vi "lua_monitor.vi"(11 "Lua for LabVIEW.lvlib:Lua.lvclass":refnum<data-value>) -> ()   [LabVIEW 2020, in "Lua for LabVIEW.lvlib" / "Lua.lvclass"]
uses:
  Lua.lvclass
  Lua.lvclass/Lua.ctl
  lib/lua.dll/lua.dll.lvlib
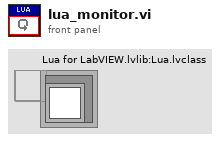
[diagram p1: front panel]
types:
  T1 = typedef "Lua for LabVIEW.lvlib/Lua.lvclass/lua_monitor_event.ctl" = enum16{"<null>", "terminate"}
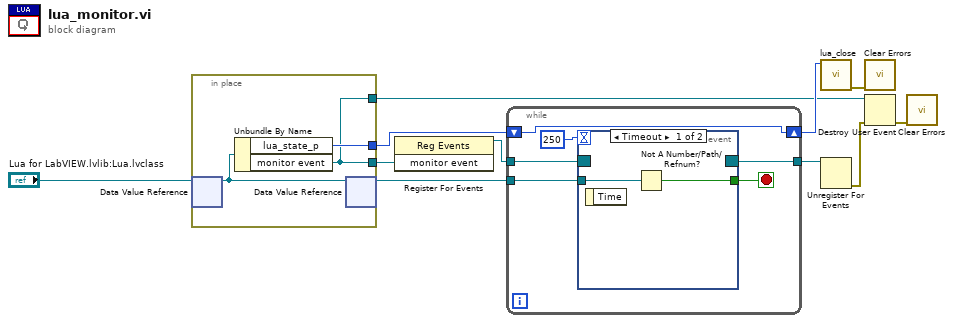
[diagram p0: block diagram]
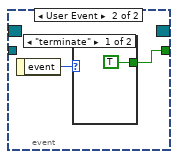
[diagram p2: hidden frame]
diagram:
  n1 = in-place {
    in-place-border: [w13] -> w8
    in-place-border: [w12] -> w2
    in-place-border: [w12] -> w7
    n2 = in-place-dvr #1("Lua for LabVIEW.lvlib:Lua.lvclass") -> (w14:refnum<class "Lua.lvclass">)  [unwired: 1 out]
    n3 = Unbundle By Name(w14) -> ("lua_state_p"=w13:u64, "monitor event"=w12:refnum<user-event>)
    n4 = in-place-dvr #1(w14) -> (w10:refnum<data-value>)  [unwired: 1 out]
  }
  n5 = register-events(w7) -> (reference out=w9:refnum<event-registration>)  [unwired: 2 in, 1 out]
  n6 = while {
    tunnel: w10 -> [w18]
    tunnel: w9 -> [w20]
    shift-right: [w16] -> w6
    shift-left: w8 -> [w16]
    tunnel: [w15] -> w4
    stop <- w17 stop-if-true
    n7 = event shown="[0] Timeout" {
      selector: w20 -> [_ _]
      dyn-events: [_ _] -> w15
      timeout: 250 -> [_ _]
      tunnel: w18 -> [w22 _]
      tunnel: [w21 w23] -> w17
      event Timeout {
        n8 = event-data() -> ()  [unwired: 1 in, 1 out]
        n9 = Not A Number/Path/Refnum?(number/path/refnum=w22) -> (NaN/Path/Refnum?=w21:bool)
      }
      event User Event {
        n10 = event-data() -> ("event"=w24:T1)  [unwired: 1 in]
        n11 = case shown="\"terminate\"" w24 {
          tunnel: [TRUE _] -> w23
          frame "terminate" {
          }
          frame Default {
          }
        }
      }
    }
  }
  n12 = call "lua_close.vi"("lua_state_p"=w6) -> ("error out"=w5:errorcluster)  [unwired: 10 in]
  n13 = Unregister For Events(event registration refnum=w4) -> (error out=w3:errorcluster)  [unwired: 1 in]
  n14 = call <vilib>:"Clear Errors.vi"("error in (no error)"=w5) -> ()  [unwired: 5 in, 2 out]
  n15 = Destroy User Event(user event=w2, error in=w3) -> (error out=w1:errorcluster)
  n16 = call <vilib>:"Clear Errors.vi"("error in (no error)"=w1) -> ()  [unwired: 5 in, 2 out]
